vi "Find SubVI.vi"(8 "error in":errorcluster, 10 "VI Path":path, 11 "VI Reference":refnum<vi>) -> (0 "error out":errorcluster, 3 "Found?":bool)   [LabVIEW 2020, in "Panther Dashboard.lvlib"]
uses:
  Panther Dashboard.lvlib
  <vilib>/Utility/traverseref.llb/TRef TravTarget.ctl
  be12010b-856d-475a-8f77-cf8d2de3ec60.vi
  <vilib>/Utility/traverseref.llb/VI Scripting - Traverse.lvlib
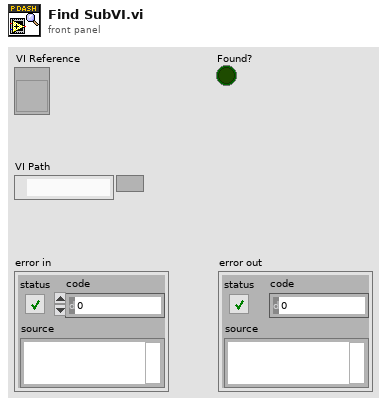
[diagram p1: front panel]
types:
  T1 = typedef "TRef TravTarget.ctl" = enum16{"FP", "BD", "Other"}
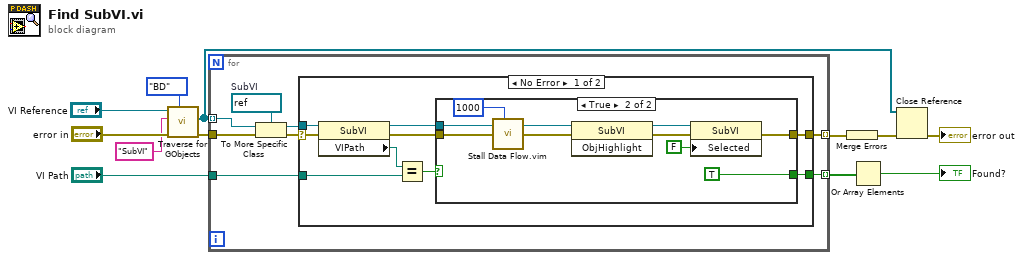
[diagram p0: block diagram]
diagram:
  n1 = call <vilib>:"Traverse for GObjects.vi"("Traverse Target"=TRef_TravTarget."BD", "error in (no error)"="error in", "Class Name"="SubVI", "VI Refnum"="VI Reference") -> ("error out"=w10:errorcluster, "References"=w3:refnum<vi>[])  [unwired: 4 in, 2 out]
  n2 = for {
    tunnel: w3 -> [w17] mode=indexing
    tunnel: "VI Path" -> [w14]
    tunnel: w10 -> [w19]
    tunnel: [w18] -> w7 mode=indexing
    tunnel: [w13] -> w2 mode=indexing
    w16 = refnum<vi> refnum  # SubVI
    n3 = To More Specific Class(target class=w16, reference=w17, error in=w19) -> (specific class reference=w15:refnum<vi>, error out=w20:errorcluster)
    n4 = case shown="No Error" w20 {
      selector: w20 -> [w28 _]
      tunnel: w15 -> [w25 _]
      tunnel: w14 -> [w22 _]
      tunnel: [w27 _] -> w18
      tunnel: [w23 _] -> w13
      frame No Error {
        n5 = property class="SubVI"(reference=w25, error in=w28) -> (reference out=w24:refnum<vi>, error out=w29:errorcluster, "VIPath"=w21:path)
        n6 = Equal?(x=w21, y=w22) -> (x = y?=w26:bool)
        n7 = case shown="True" w26 {
          tunnel: w24 -> [_ w36]
          tunnel: w29 -> [w30 w37]
          tunnel: [w30 w38] -> w27
          tunnel: [_ TRUE ("Selected")] -> w23
          frame False {
          }
          frame True {
            n8 = call "Stall Data Flow.vim"("value in"=w37, "milliseconds to wait"=u32 1000) -> ("value out"=w32:errorcluster)  [unwired: 1 out]
            n9 = invoke class="SubVI" method="ObjHighlight"(reference=w36, error in=w32) -> (reference out=w35:refnum<vi>, error out=w39:errorcluster)  [unwired: 1 in, 1 out]
            n10 = property class="SubVI"(reference=w35, error in=w39, "Selected"=FALSE) -> (error out=w38:errorcluster)  [unwired: 1 out]
          }
        }
      }
      frame Error {
      }
    }
  }
  n11 = Merge Errors(w7) -> (w11:errorcluster)
  n12 = Or Array Elements(Boolean array=w2) -> (logical OR=→"Found?":bool)
  n13 = Close Reference(reference=w3, error in (no error)=w11) -> (error out=→"error out":errorcluster)
